vi "Custom Name.vi"(10 "Pattern Part":T1) -> (2 "Custom Name?":bool)   [LabVIEW 2020, in "Stream.lvlib" / "URLPattern.lvclass"]
uses:
  URLPattern.lvclass
  Pattern Part.ctl
  Pattern Part Type.ctl
  Pattern Part Modifier.ctl
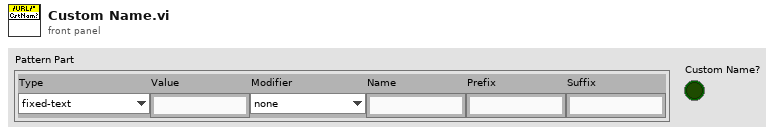
[diagram p1: front panel]
types:
  T1 = typedef "Stream.lvlib/URLPattern.lvclass/Pattern Part.ctl" = cluster{"Type":T2, "Value":string, "Modifier":T3, "Name":string, "Prefix":string, "Suffix":string}
  T2 = typedef "Stream.lvlib/URLPattern.lvclass/Pattern Part Type.ctl" = enum16{"fixed-text", "regexp", "segment-wildcard", "full-wildcard"}
  T3 = typedef "Stream.lvlib/URLPattern.lvclass/Pattern Part Modifier.ctl" = enum16{"none", "optional", "zero-or-more", "one-or-more"}
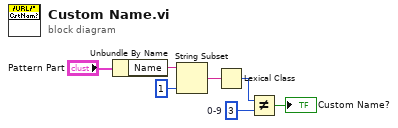
[diagram p0: block diagram]
diagram:
  w2 = i16 3  # 0-9
  n1 = Unbundle By Name("Pattern Part") -> ("Name"=w6:string)
  n2 = String Subset(string=w6, length (rest)=1 ("length (rest)")) -> (substring=w4:string)  [unwired: 1 in]
  n3 = Lexical Class(1:w4) -> (0:w3:i16)
  n4 = Not Equal?(x=w3, y=w2) -> (x != y?=→"Custom Name?":bool)
